vi "Enable_TCU.vi"() -> (0 "error out":errorcluster)   [LabVIEW 2018]
uses:
  SupportVIs/VISA Configure Serial Port (Instr).vi
panel:
  in  "error in (no error)":errorcluster
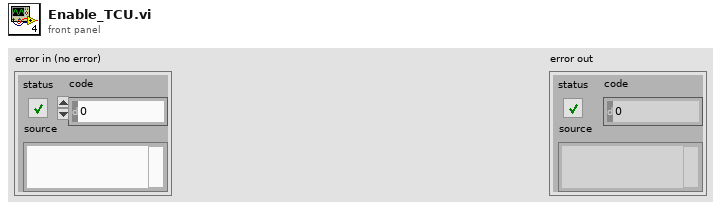
[diagram p1: front panel]
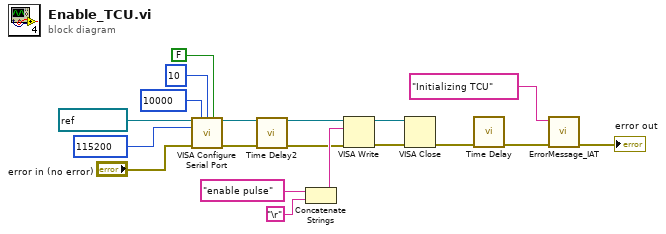
[diagram p0: block diagram]
diagram:
  n1 = call-poly "VISA Configure Serial Port"("VISA resource name"=refnum<visa-resource-name> "COM3", "timeout (10sec)"=u32 10000, "termination char\n(0xA = '\\n' = LF)"=u8 10 ("termination char\n(0xA = '\\n' = LF)"), "Enable Termination\nChar (T)"=FALSE ("Enable Termination\nChar (T)"), "baud rate (9600)"=u32 115200, "error in (no error)"="error in (no error)") -> ("VISA resource name out"=w7:refnum<visa-resource-name>, "error out"=w9:errorcluster)  [unwired: 8 in]
  n2 = call "Time Delay2"("error in (no error)"=w9) -> ("error out"=w8:errorcluster)  [unwired: 10 in]
  n3 = Concatenate Strings("enable pulse" ("write buffer"), "\r") -> (w14:string)
  n4 = VISA Write(VISA resource name=w7, write buffer=w14, error in (no error)=w8) -> (VISA resource name out=w12:refnum<visa-resource-name>, error out=w11:errorcluster)  [unwired: 1 out]
  n5 = VISA Close(VISA resource name=w12, error in (no error)=w11) -> (error out=w10:errorcluster)
  n6 = call "Time Delay"("error in (no error)"=w10) -> ("error out"=w2:errorcluster)  [unwired: 10 in]
  n7 = call "ErrorMessage_IAT.vi"("error in (no error)"=w2, "Message"="Initializing TCU") -> ("error out"=→"error out":errorcluster)  [unwired: 9 in]
